vi "Transfer Item - File Transfer Factory - Get.vi"(4 "Remove Origin":bool, 6 "RemotePath":string, 7 "Transfer Type":T4, 8 "error in (no error)":errorcluster, 9 "LocalPath":string, 10 "Transfer Options":refnum<class "FileTransferOptions.lvclass">, 11 "Session in":refnum<class "Session.lvclass">) -> (0 "error out":errorcluster, 2 "Transfer Status":T3)   [LabVIEW 2015, in "LV-WinSCP.lvlib"]
uses:
  Transfer Type.ctl
  Classes/FileTransferOptions/FileTransferOptions.lvclass
  Classes/Session/Session.lvclass
  Classes/FileTransfer/FileAndDestination.ctl
  Classes/FileTransfer/TransferExceptionDescription.ctl
  Classes/FileTransfer/TransferFiles-Get/TransferFiles-Get.lvclass
  Classes/FileTransfer/TransferFolder-Get/TransferFolder-Get.lvclass
  Classes/FileTransfer/FileTransfer.lvclass
  LV-WinSCP.lvlib
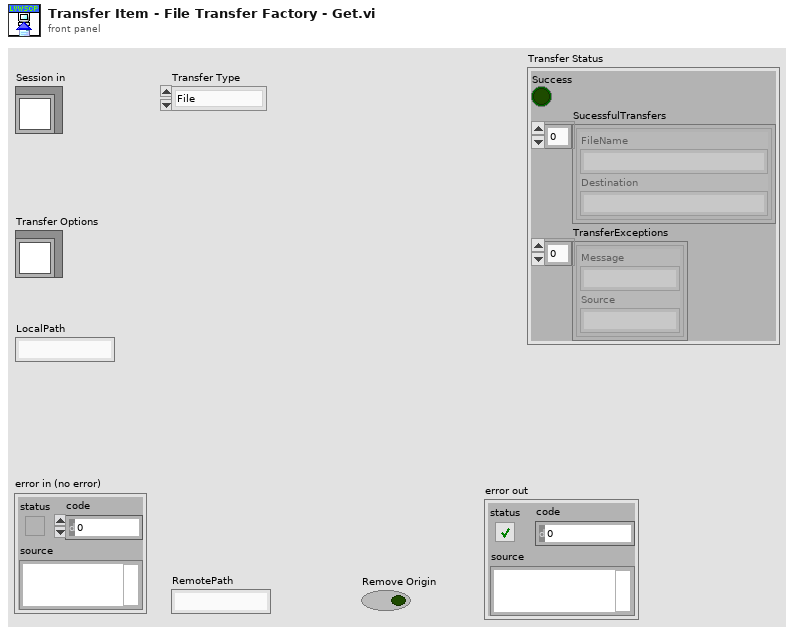
[diagram p1: front panel]
types:
  T1 = typedef "WinSCP.lvlib/FileTransfer.lvclass/FileAndDestination.ctl" = cluster{"FileName":string, "Destination":string}
  T2 = typedef "WinSCP.lvlib/FileTransfer.lvclass/TransferExceptionDescription.ctl" = cluster{"Message":string, "Source":string}
  T3 = cluster{"Success":bool, "SucessfulTransfers":T1[], "TransferExceptions":T2[]}
  T4 = typedef "LV-WinSCP.lvlib/Transfer Type.ctl" = enum16{"File", "Folder"}
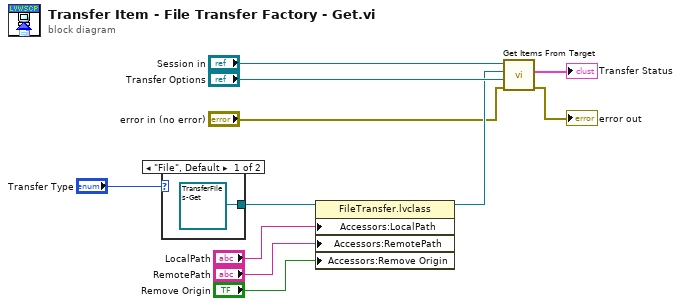
[diagram p0: block diagram]
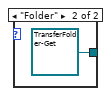
[diagram p2: hidden frame]
diagram:
  n1 = case shown="\"File\", Default" "Transfer Type" {
    tunnel: [refnum<class "TransferFiles-Get.lvclass"> refnum ("WinSCP.lvlib:TransferFiles-Get.lvclass") refnum<class "TransferFolder-Get.lvclass"> refnum ("WinSCP.lvlib:TransferFolder.lvclass")] -> w7
    frame "File", Default {
    }
    frame "Folder" {
    }
  }
  n2 = property class="FileTransfer.lvclass"(reference=w7, "Accessors:LocalPath"="LocalPath", "Accessors:RemotePath"="RemotePath", "Accessors:Remove Origin"="Remove Origin") -> (reference out=w6:refnum<class "FileTransfer.lvclass">)  [unwired: 1 in, 1 out]
  n3 = call-dynamic "Get Items From Target.vi"("error in (no error)"="error in (no error)", "Transfer Options"="Transfer Options", "FileTransfer"=w6, "Session in"="Session in") -> ("error out"=→"error out":errorcluster, "Transfer Status"=→"Transfer Status":T3)  [unwired: 5 in, 1 out]
